vi "AO_2Chan.vi"() -> ()   [LabVIEW 2021]
doc: "This example demonstrates how to generate a user-defined voltage using the analog output of a DAQ device."
uses:
  <vilib>/Utility/error.llb/DialogType.ctl
  <vilib>/DAQmx/write.llb/DAQmx Write (Analog 1D DBL NChan 1Samp).vi
  <vilib>/DAQmx/create/channels.llb/DAQmx Create Channel (AO-Voltage-Basic).vi
  <vilib>/DAQmx/miscellaneous.llb/DAQmx Fill In Error Info.vi
panel:
  in  "Tab Control":enum32{"Manual", "Toggle"}(tab)
  in  "Control":enum16{"Up", "Zero", "Down"}[](array[ring])
  out "Output":dbl[](array[numeric])
  in  "Pulse Width":u32=100
  in  "Stop":bool
  in  "Max Voltage":dbl=10.0
  in  "Min Voltage":dbl=-10.0
  in  "Physical Channel(s)":tag="Dev2/ao0:1"
  # "Channel Settings"
  # "Output"
  # "The number of elements in the channel array\nmust equal the number of channels in the task."
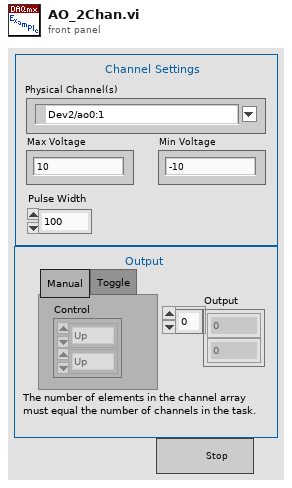
[diagram p1: front panel]
types:
  T1 = typedef "DialogType.ctl" = u16
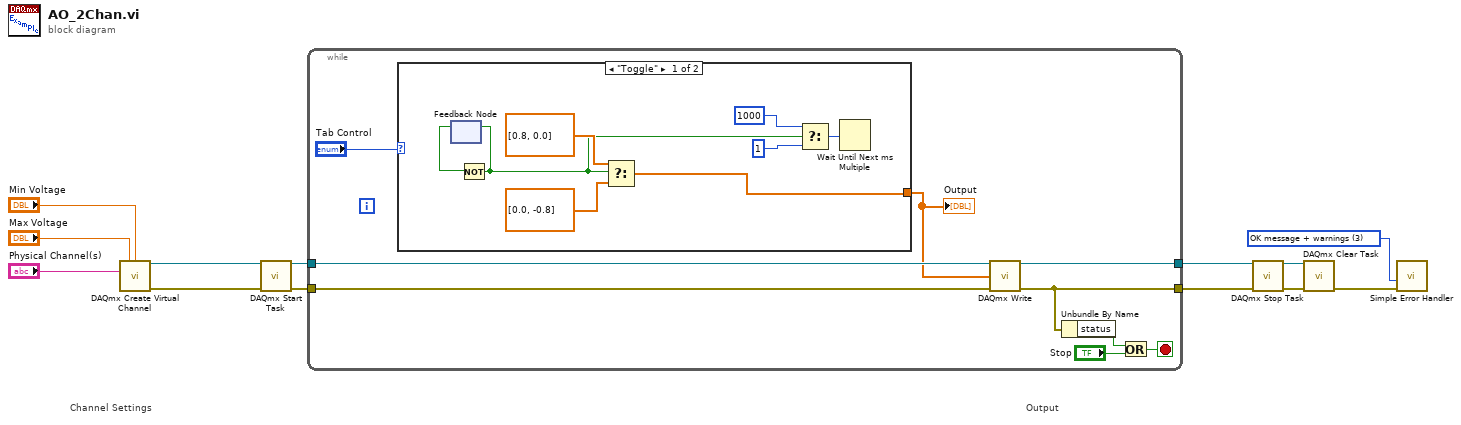
[diagram p0: block diagram]
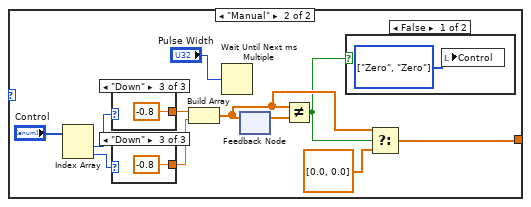
[diagram p2: hidden frame]
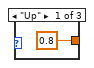
[diagram p4: hidden frame]
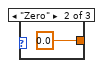
[diagram p5: hidden frame]
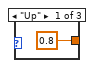
[diagram p6: hidden frame]
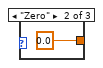
[diagram p7: hidden frame]
diagram:
  w1 = T1 3 items=["no dialog", "OK message", "continue or stop message", "OK message + warnings", "continue/stop + warnings"] ("type of dialog (OK msg:1)")
  # "Output"
  # "Channel Settings"
  n1 = call-poly <vilib>:"DAQmx Create Virtual Channel.vi"("maximum value"="Max Voltage", "minimum value"="Min Voltage", "physical channels"="Physical Channel(s)") -> ("task out"=w9:refnum<k21>, "error out"=w8:errorcluster)  [unwired: 11 in]
  n2 = call <vilib>:"DAQmx Start Task.vi"("task/channels in"=w9, "error in"=w8) -> ("task out"=w7:refnum<k21>, "error out"=w6:errorcluster)  [unwired: 12 in]
  n3 = while {
    tunnel: w7 -> [w22]
    tunnel: w6 -> [w21]
    tunnel: [w17] -> w4
    tunnel: [w20] -> w5
    stop <- w16 stop-if-true
    n4 = case shown="\"Toggle\"" "Tab Control" {
      tunnel: [w27 w39] -> w15
      frame "Toggle" {
        n5 = feedback #1() -> (w28:bool)  [unwired: 1 in]
        n6 = Not(x=w28) -> (.not. x?=w23:bool)
        n7 = feedback-in #1(w23) -> ()
        n8 = Select(t=dbl[] [0.8, 0.0] ("f"), s=w23, f=dbl[] [0.0, -0.8]) -> (s? t:f=w27:dbl[])
        n9 = Select(t=u32 1000 ("Pulse Width"), s=w23, f=u32 1 ("Pulse Width")) -> (s? t:f=w26:u32)
        n10 = Wait Until Next ms Multiple(millisecond multiple=w26) -> ()  [unwired: 1 out]
      }
      frame "Manual" {
        n11 = Index Array(array="Control") -> (element #1=w37:enum16{"Up", "Zero", "Down"}, element #2=w35:enum16{"Up", "Zero", "Down"})  [unwired: 2 in]
        n12 = case shown="\"Down\"" w37 {
          tunnel: [0.8 0.0 -0.8] -> w36
          frame "Up" {
          }
          frame "Zero" {
          }
          frame "Down" {
          }
        }
        n13 = case shown="\"Down\"" w35 {
          tunnel: [0.8 0.0 -0.8] -> w34
          frame "Up" {
          }
          frame "Zero" {
          }
          frame "Down" {
          }
        }
        n14 = Build Array(w36, w34) -> (w33:dbl[])
        n15 = Wait Until Next ms Multiple(millisecond multiple="Pulse Width") -> ()  [unwired: 1 out]
        n16 = feedback #2() -> (w41:dbl[])  [unwired: 1 in]
        n17 = feedback-in #2(w33) -> ()
        n18 = Not Equal?(x=w33, y=w41) -> (x != y?=w32:bool)
        n19 = case shown="False" w32 {
          frame False {
            w42 = enum16{"Up", "Zero", "Down"}[] [enum."Zero", enum."Zero"] items=["Up", "Zero", "Down"] ("Control")
            n20 = local write "Control"(w42) -> ()
          }
          frame True {
          }
        }
        n21 = Select(t=w33, s=w32, f=dbl[] [0.0, 0.0]) -> (s? t:f=w39:dbl[])
      }
    }
    "Output" <- w15
    n22 = call-poly <vilib>:"DAQmx Write.vi"("task/channels in"=w22, "data"=w15, "error in"=w21) -> ("task out"=w20:refnum<k21>, "error out"=w17:errorcluster)  [unwired: 10 in, 1 out]
    n23 = Unbundle By Name(w17) -> ("status"=w19:bool)
    n24 = Or(x=w19, y="Stop") -> (x .or. y?=w16:bool)
  }
  n25 = call <vilib>:"DAQmx Stop Task.vi"("task/channels in"=w5, "error in"=w4) -> ("task out"=w3:refnum<k21>, "error out"=w2:errorcluster)  [unwired: 12 in]
  n26 = call <vilib>:"DAQmx Clear Task.vi"("task in"=w3, "error in"=w2) -> ("error out"=w13:errorcluster)  [unwired: 13 in]
  n27 = call <vilib>:"Simple Error Handler.vi"("type of dialog (OK msg:1)"=w1, "error in (no error)"=w13) -> ()  [unwired: 3 in, 5 out]
